vi "Polarisation.vi"(0 "VISA resource name":refnum<visa-resource-name>, 3 "Shutter Ctrls 2":refnum<vi>, 6 "Shutter on?":bool, 7 "ESP301 Error":errorcluster, 8 "LightField Automation in":refnum<class "LightField Automation.lvclass">, 9 "RotStage Exc Angle Refnum":refnum<vi>, 10 "KCube Shutter Device Reference 2":refnum<vi>, 11 "StopPolar 2":refnum<vi>, 12 "CCD 1D Spectrum Main 3":refnum<vi>, 13 "LightField error":errorcluster, 14 "Polar Params SubVI":T2, 15 "PausePolar":refnum<vi>, 17 "Axis ESP301 / RotStage":u16(ring) items=["RotStage Detection"=2, "RotStage Excitation"=3], 21 "IntGraph Refnum":refnum<vi>, 24 "Slide Refnum":refnum<vi>) -> (2 "KCube Shutter Device Reference":refnum<k24>, 18 "Angles":dbl[](array[numeric]), 19 "Wavelengths":dbl[](array[numeric]), 20 "VISA resource name out":refnum<visa-resource-name>, 23 "LightField Automation out":refnum<class "LightField Automation.lvclass">, 25 "LightField error out":errorcluster, 26 "2D Pol Data":dbl[][](array[numeric]), 27 "ESP301 Error out":errorcluster)   [LabVIEW 2019]
uses:
  Light Field/lightfield-automation-labview/LightField Automation.lvclass
  TypeDefs/AcqMode.ctl
  D:/Users/manip-thz/Documents/Controle_Manip_2020/Thorlabs.MotionControl.KCube.SolenoidCLI.dll
  Thorlabs.MotionControl.KCube.SolenoidCLI.dll
  Newport/Newport ESP301/Newport ESP301.lvlib
panel:
  in  "Polar mode":u16(ring)=3 caption="Rotate HWP" items=["Excitation"=3, "Detection"=2]
  in  "Previous Button":bool
  in  "StopPolar":bool
  out "CCD 1D Spectrum Main 2":cluster{dbl[], dbl[]}(graph)
  in  "XYGraph Refnum":refnum<vi>
  in  "Acq Mode":T1=enum."Spectrum" caption="Acq mode"
  out "2D Data":dbl[][](array[numeric])
  in  "RotStage Exc Angle (°)":dbl=2.0 caption="Readout (°)" min=-360.0 max=360.0
  out "Position (units)":dbl format="%.6g"
  out "Numeric":i32
  out "Motion Done":bool
  in  "Progress":u8(slide) scale=0.0..100.0
  out "Current angle (°)":dbl
  in  "CCD ROI":T3(ring)
  in  "Exposure time (ms)":dbl=100.0
  in  "Step Angle (°)":dbl=5.0
  in  "End Angle (°)":dbl=180.0
  in  "Start Angle (°)":dbl
types:
  T1 = typedef "AcqMode.ctl" = enum16{"Image", "Spectrum", "APD 1", "APD 2", "APD 1+2"}
  T2 = cluster{"Polar End Angle (°)":dbl, "Polar Start Angle (°)":dbl, "Polar Step Angle (°)":dbl, "Acq Mode":T1, "Polar mode":u16, "Exposure Time (ms)":dbl, "CCD ROI":enum16{"Custom ROI", "Full sensor", "Binned full sensor"}}
  T3 = enum16{"Custom ROI", "Full sensor", "Binned full sensor"}
  T4 = enum16{"Contrast", "Spectre", "Polarisation", "Time Trace", "XY Intensity Map"}
  T5 = cluster{"Image":dbl[][][], "Frame Size":cluster{"F":i32, "Y":i32, "X":i32}}[]
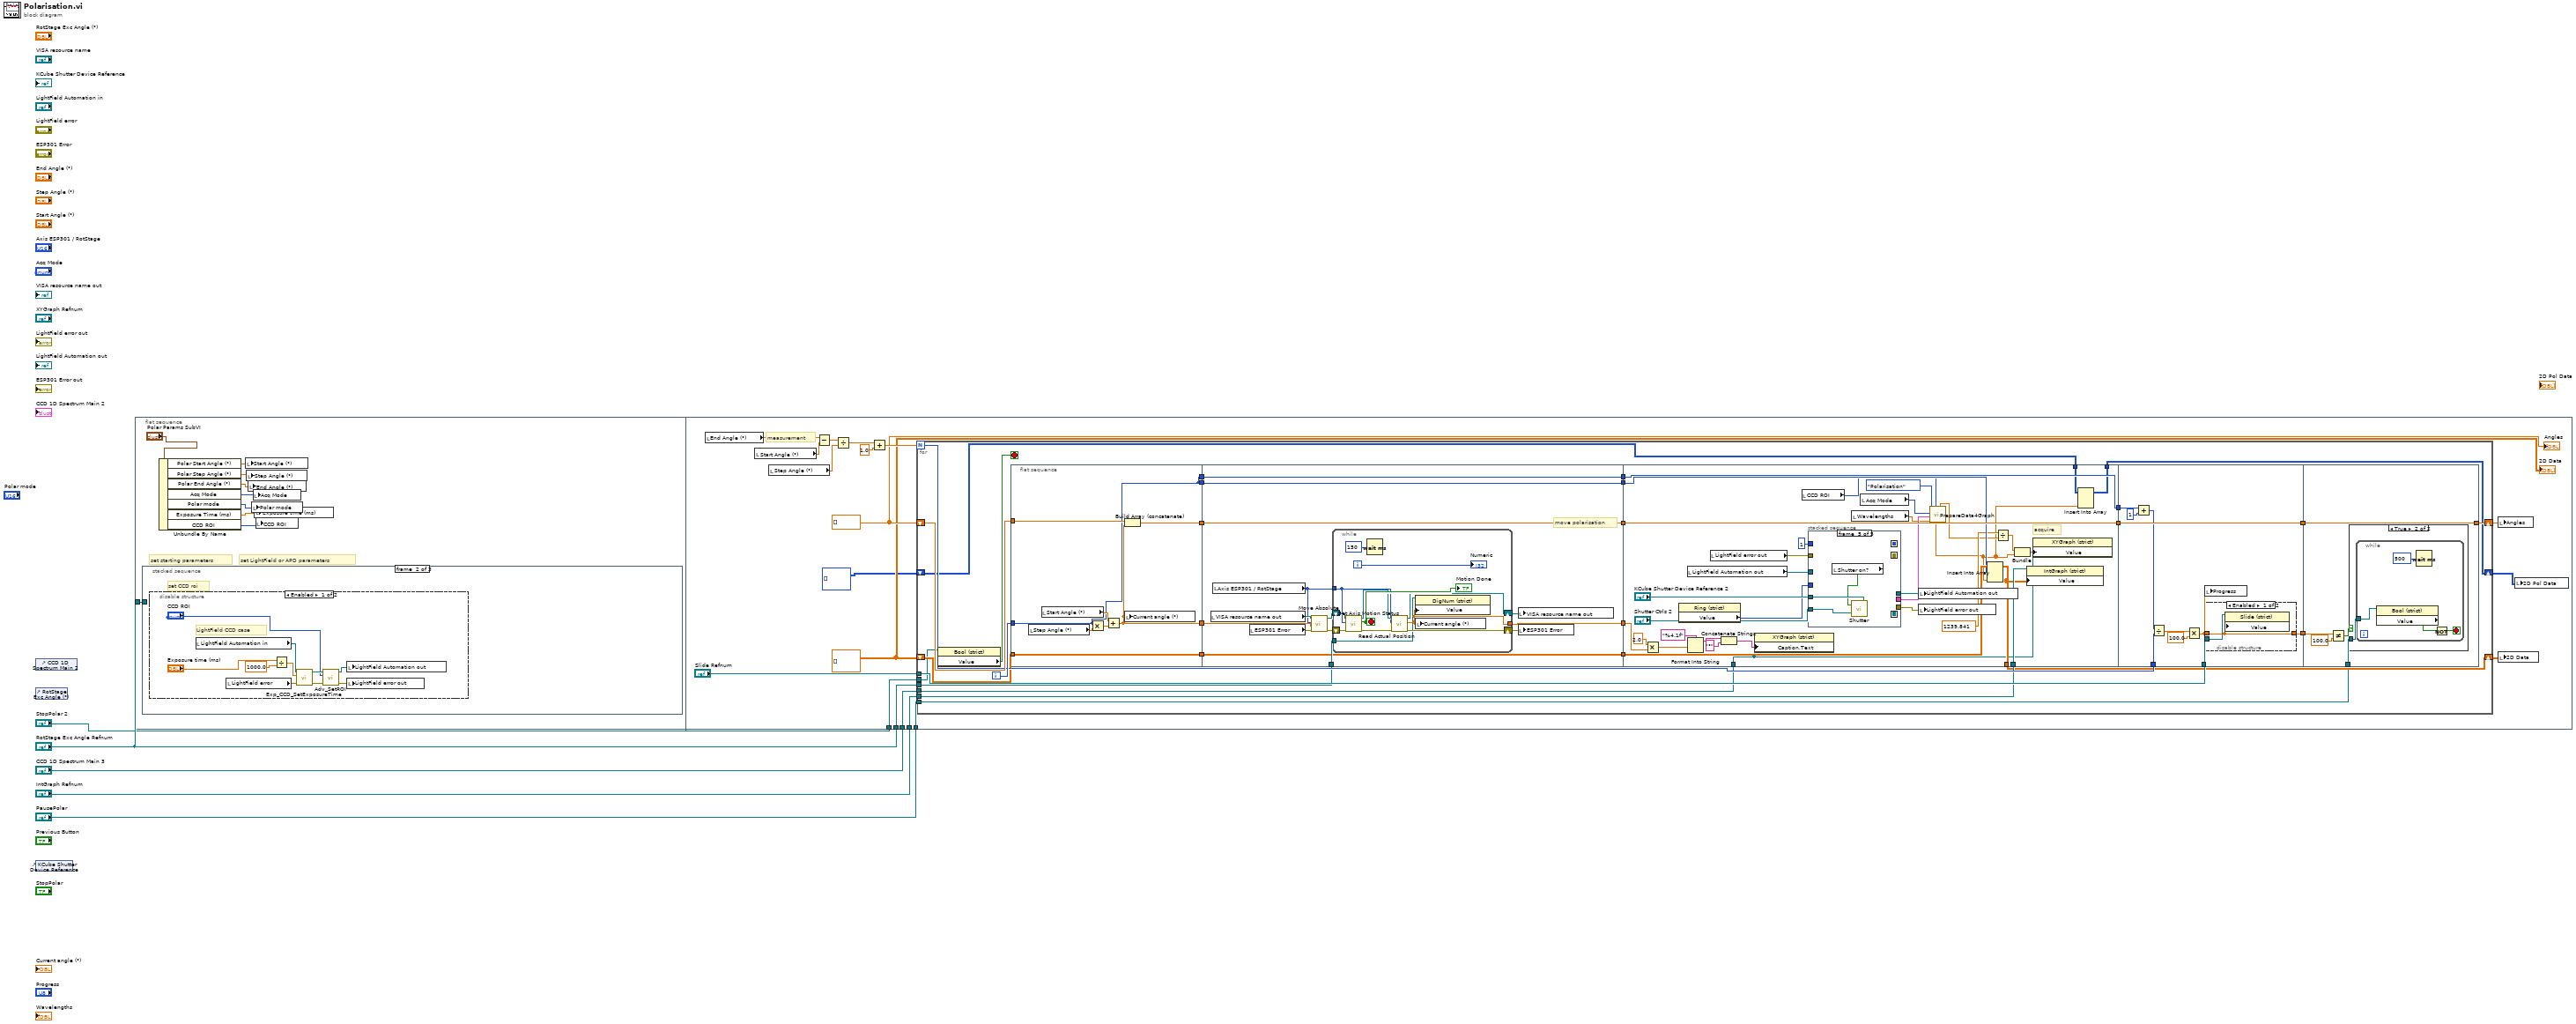
[diagram p0: block diagram]
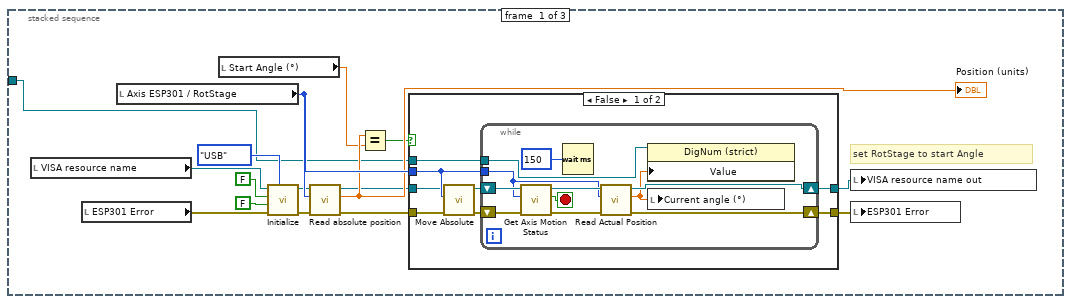
[diagram p2: hidden frame]
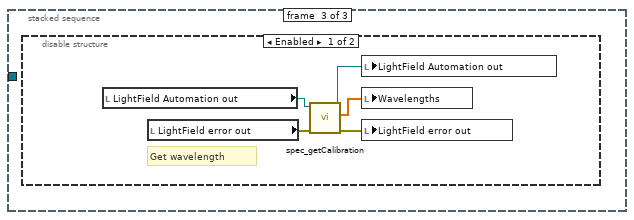
[diagram p5: hidden frame]
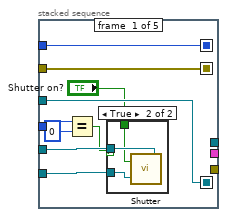
[diagram p7: hidden frame]
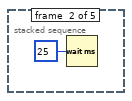
[diagram p9: hidden frame]
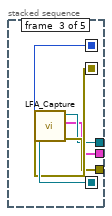
[diagram p10: hidden frame]
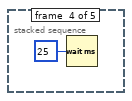
[diagram p11: hidden frame]
diagram:
  n1 = control-ref of="CCD 1D Spectrum Main 2"() -> ()  [unwired: 1 out]
  n2 = control-ref of="RotStage Exc Angle (°)"() -> ()  [unwired: 1 out]
  n3 = control-ref of="KCube Shutter Device Reference"() -> ()  [unwired: 1 out]
  n4 = flat-sequence {
    tunnel: "RotStage Exc Angle Refnum" -> [w14]
    tunnel: "RotStage Exc Angle Refnum" -> [w75]
    tunnel: "IntGraph Refnum" -> [w74]
    tunnel: "CCD 1D Spectrum Main 3" -> [w71]
    tunnel: "StopPolar 2" -> [w70]
    tunnel: "PausePolar" -> [w69]
    frame #0 {
      # "set LightField or APD parameters"
      # "set starting parameters"
      n5 = stacked-sequence {
        tunnel: w14 -> [w15 _ _]
        frame #0 {
          # "set RotStage to start Angle"
          n6 = local read "VISA resource name"() -> (w22:refnum<visa-resource-name>)
          n7 = local read "ESP301 Error"() -> (w16:errorcluster)
          n8 = local read "Axis ESP301 / RotStage"() -> (w28:u16)
          n9 = local read "Start Angle (°)"() -> (w26:dbl)
          n10 = call "Initialize.vi"("VISA resource name"=w22, "ID Query (True)"=FALSE, "Reset (False)"=FALSE, "error in (no error)"=w16, "Serial Link (RS232)"=enum16{"RS232", "USB"}."USB") -> ("VISA resource name out"=w18:refnum<visa-resource-name>, "error out"=w17:errorcluster)  [unwired: 4 in]
          n11 = call "Read absolute position.vi"("error in (no error)"=w17, "Axis (1)"=w28, "VISA resource name"=w18) -> ("error out"=w24:errorcluster, "Position (units)"=w27:dbl, "VISA resource name out"=w23:refnum<visa-resource-name>)  [unwired: 2 in]
          "Position (units)" <- w27
          n12 = Equal?(x=w27, y=w26) -> (x = y?=w25:bool)
          n13 = case shown="False" w25 {
            tunnel: [w38 w51] -> w30
            tunnel: [w37 w50] -> w29
            tunnel: w28 -> [w34 _]
            tunnel: w24 -> [w33 w50]
            tunnel: w23 -> [w32 w51]
            tunnel: w15 -> [w31 _]
            frame False {
              n14 = call "Move Absolute.vi"("error in (no error)"=w33, "Axis (1)"=w34, "VISA resource name"=w32) -> ("error out"=w35:errorcluster, "VISA resource name out"=w36:refnum<visa-resource-name>)  [unwired: 3 in]
              n15 = while {
                tunnel: w34 -> [w43]
                shift-right: [w44] -> w38
                shift-left: w36 -> [w49]
                shift-right: [w41] -> w37
                shift-left: w35 -> [w48]
                tunnel: w31 -> [w39]
                stop <- w47 stop-if-true
                n16 = call "Get Axis Motion Status.vi"("error in (no error)"=w48, "Axis (1)"=w43, "VISA resource name"=w49) -> ("error out"=w42:errorcluster, "Motion Done"=w47:bool, "VISA resource name out"=w45:refnum<visa-resource-name>)  [unwired: 2 in]
                n17 = Wait (ms)(milliseconds to wait=u32 150) -> ()  [unwired: 1 out]
                n18 = call "Read Actual Position.vi"("error in (no error)"=w42, "Axis (1)"=w43, "VISA resource name"=w45) -> ("error out"=w41:errorcluster, "Position (units)"=w40:dbl, "VISA resource name out"=w44:refnum<visa-resource-name>)  [unwired: 2 in]
                n19 = property class="DigNum (strict)"(reference=w39, "Value"=w40) -> ()  [unwired: 1 in, 2 out]
                n20 = local write "Current angle (°)"(w40) -> ()
              }
            }
            frame True {
            }
          }
          n21 = local write "VISA resource name out"(w30) -> ()
          n22 = local write "ESP301 Error"(w29) -> ()
        }
        frame #1 {
          # "set CCD roi"
          n23 = disable-structure shown="Enabled" {
            frame Enabled {
              # "LightField CCD case"
              n24 = local read "LightField Automation in"() -> (w57:refnum<class "LightField Automation.lvclass">)
              n25 = local read "LightField error"() -> (w58:errorcluster)
              n26 = Divide(x="Exposure time (ms)", y=1000.0) -> (x/y=w59:dbl)
              n27 = call "Exp_CCD_SetExposureTime.vi"("error in (no error)"=w58, "Exposure Time (s)"=w59, "LightField Automation in"=w57) -> ("error out"=w55:errorcluster, "LightField Automation out"=w56:refnum<class "LightField Automation.lvclass">)  [unwired: 7 in]
              n28 = call "Adv_SetROI.vi"("error in (no error)"=w55, "ROI"="CCD ROI", "LightField Automation in"=w56) -> ("error out"=w54:errorcluster, "LightField Automation out"=w53:refnum<class "LightField Automation.lvclass">)  [unwired: 7 in]
              n29 = local write "LightField Automation out"(w53) -> ()
              n30 = local write "LightField error out"(w54) -> ()
            }
            frame Disabled {
            }
          }
        }
        frame #2 {
          n31 = disable-structure shown="Enabled" {
            frame Enabled {
              # "Get wavelength"
              n32 = local read "LightField Automation out"() -> (w66:refnum<class "LightField Automation.lvclass">)
              n33 = local read "LightField error out"() -> (w65:errorcluster)
              n34 = call "spec_getCalibration.vi"("error in (no error)"=w65, "LightField Automation in"=w66) -> ("error out"=w63:errorcluster, "ColumnCalibration"=w62:dbl[], "LightField Automation out"=w64:refnum<class "LightField Automation.lvclass">)  [unwired: 7 in]
              n35 = local write "LightField Automation out"(w64) -> ()
              n36 = local write "Wavelengths"(w62) -> ()
              n37 = local write "LightField error out"(w63) -> ()
            }
            frame Disabled {
            }
          }
        }
      }
      n38 = Unbundle By Name("Polar Params SubVI") -> ("Polar Start Angle (°)"=w10:dbl, "Polar Step Angle (°)"=w11:dbl, "Polar End Angle (°)"=w9:dbl, "Acq Mode"=w8:T1, "Polar mode"=w6:u16, "Exposure Time (ms)"=w7:dbl, "CCD ROI"=w12:T3)
      n39 = local write "Start Angle (°)"(w10) -> ()
      n40 = local write "Step Angle (°)"(w11) -> ()
      n41 = local write "End Angle (°)"(w9) -> ()
      n42 = local write "Polar mode"(w6) -> ()
      n43 = local write "Acq Mode"(w8) -> ()
      n44 = local write "Exposure time (ms)"(w7) -> ()
      n45 = local write "CCD ROI"(w12) -> ()
    }
    frame #1 {
      w73 = dbl[][] []
      w76 = dbl[] []
      # "measurement"
      n46 = local read "End Angle (°)"() -> (w78:dbl)
      n47 = local read "Start Angle (°)"() -> (w79:dbl)
      n48 = local read "Step Angle (°)"() -> (w81:dbl)
      n49 = Subtract(x=w78, y=w79) -> (x-y=w80:dbl)
      n50 = Divide(x=w80, y=w81) -> (x/y=w82:dbl)
      n51 = Add(x=w82, y=1.0) -> (x+y=w83:dbl)
      n52 = for {
        N: w83 -> [w110]
        shift-right: [w113] -> w84
        shift-left: w76 -> [w114]
        tunnel: "Slide Refnum" -> [w108]
        tunnel: w75 -> [w102]
        tunnel: w74 -> [w101]
        shift-right: [w97] -> w72
        shift-left: w73 -> [w100]
        tunnel: w71 -> [w94]
        tunnel: w70 -> [w92]
        tunnel: w69 -> [w89]
        shift-right: [w86] -> w67
        shift-left: i32[][] [] -> [w87]
        i -> [w112]
        stop <- w91 stop-if-true
        n53 = property class="Bool (strict)"(reference=w92) -> ("Value"=w91:bool)  [unwired: 1 in, 2 out]
        n54 = flat-sequence {
          tunnel: w114 -> [w122]
          tunnel: w112 -> [w115]
          tunnel: [w121] -> w107
          tunnel: [w115] -> w105
          tunnel: [w117] -> w103
          tunnel: w100 -> [w116]
          tunnel: [w116] -> w98
          tunnel: [w115] -> w96
          tunnel: w107 -> [w136]
          tunnel: [w136] -> w106
          tunnel: w105 -> [w135]
          tunnel: [w135] -> w104
          tunnel: w103 -> [w132]
          tunnel: w102 -> [w126]
          tunnel: [w125] -> w99
          tunnel: w98 -> [w125]
          tunnel: w96 -> [w124]
          tunnel: [w124] -> w95
          tunnel: [w123] -> w93
          tunnel: w106 -> [w179]
          tunnel: [w179] -> w111
          tunnel: [w182] -> w109
          tunnel: w104 -> [w182]
          tunnel: w101 -> [w181]
          tunnel: w99 -> [w180]
          tunnel: [w178] -> w97
          tunnel: w95 -> [w177]
          tunnel: w94 -> [w168]
          tunnel: w93 -> [w158]
          tunnel: w87 -> [w154]
          tunnel: [w153] -> w86
          tunnel: w111 -> [w215]
          tunnel: w110 -> [w212]
          tunnel: w109 -> [w211]
          tunnel: w108 -> [w208]
          tunnel: [w215] -> w90
          tunnel: [w206] -> w88
          tunnel: [w222] -> w113
          tunnel: w90 -> [w222]
          tunnel: w89 -> [w221]
          tunnel: w88 -> [w220]
          frame #0 {
            n55 = local read "Step Angle (°)"() -> (w119:dbl)
            n56 = local read "Start Angle (°)"() -> (w120:dbl)
            n57 = Multiply(x=w115, y=w119) -> (x*y=w118:dbl)
            n58 = Add(x=w120, y=w118) -> (x+y=w117:dbl)
            n59 = Build Array (concatenate)(w122, w117) -> (w121:dbl[])
            n60 = local write "Current angle (°)"(w117) -> ()
          }
          frame #1 {
            # "move polarisation"
            n61 = local read "VISA resource name out"() -> (w134:refnum<visa-resource-name>)
            n62 = local read "Axis ESP301 / RotStage"() -> (w129:u16)
            n63 = local read "ESP301 Error"() -> (w133:errorcluster)
            n64 = call "Move Absolute.vi"("error in (no error)"=w133, "Position (0 units)"=w132, "Axis (1)"=w129, "VISA resource name"=w134) -> ("error out"=w131:errorcluster, "VISA resource name out"=w130:refnum<visa-resource-name>)  [unwired: 2 in]
            n65 = while {
              tunnel: w129 -> [w141]
              shift-right: [w140] -> w127
              shift-left: w130 -> [w146]
              shift-right: [w139] -> w128
              shift-left: w131 -> [w147]
              tunnel: w126 -> [w138]
              tunnel: [w137] -> w123
              i -> [w145]
              stop <- w148 stop-if-true
              n66 = call "Get Axis Motion Status.vi"("error in (no error)"=w147, "Axis (1)"=w141, "VISA resource name"=w146) -> ("error out"=w143:errorcluster, "Motion Done"=w148:bool, "VISA resource name out"=w142:refnum<visa-resource-name>)  [unwired: 2 in]
              "Motion Done" <- w148
              n67 = Wait (ms)(milliseconds to wait=u32 150) -> ()  [unwired: 1 out]
              n68 = call "Read Actual Position.vi"("error in (no error)"=w143, "Axis (1)"=w141, "VISA resource name"=w142) -> ("error out"=w139:errorcluster, "Position (units)"=w137:dbl, "VISA resource name out"=w140:refnum<visa-resource-name>)  [unwired: 2 in]
              n69 = property class="DigNum (strict)"(reference=w138, "Value"=w137) -> ()  [unwired: 1 in, 2 out]
              n70 = local write "Current angle (°)"(w137) -> ()
              "Numeric" <- w145
            }
            n71 = local write "VISA resource name out"(w127) -> ()
            n72 = local write "ESP301 Error"(w128) -> ()
          }
          frame #2 {
            # "acquire"
            n73 = Multiply(x=2.0, y=w158) -> (x*y=w160:dbl)
            n74 = property class="Ring (strict)"(reference="Shutter Ctrls 2") -> ("Value"=w155:u16)  [unwired: 1 in, 2 out]
            n75 = local read "LightField Automation out"() -> (w176:refnum<class "LightField Automation.lvclass">)
            n76 = Format Into String(format string="%4.1f", w160) -> (resulting string=w167:string)  [unwired: 2 in, 1 out]
            n77 = local read "LightField error out"() -> (w175:errorcluster)
            n78 = Concatenate Strings(w167, "°") -> (w165:string)
            n79 = property class="XYGraph (strict)"(reference=w168, "Caption.Text"=w165) -> ()  [unwired: 1 in, 2 out]
            n80 = local read "CCD ROI"() -> (w149:T3)
            n81 = stacked-sequence {
              seq-local: [w191 _ _ _ _] -> [_ _ w201 _ _]
              seq-local: [w190 _ _ _ _] -> [_ _ w200 _ _]
              seq-local: [w189 _ _ _ _] -> [_ _ w196 _ _]
              tunnel: w176 -> [w191 _ _ _ _]
              tunnel: w175 -> [w190 _ _ _ _]
              tunnel: 1 ("Frames") -> [w189 _ _ _ _]
              tunnel: [_ _ w199 _ _] -> w174
              tunnel: [_ _ w198 _ _] -> w173
              tunnel: [_ _ w197 _ _] -> w172
              tunnel: "Shutter Ctrls 2" -> [w187 _ _ _ w205]
              tunnel: "KCube Shutter Device Reference 2" -> [w188 _ _ _ w204]
              tunnel: w155 -> [w186 _ _ _ _]
              frame #0 {
                n82 = Equal?(x=w186, y=u16 0) -> (x = y?=w185:bool)
                n83 = case shown="True" w185 {
                  tunnel: w188 -> [_ w194]
                  tunnel: w187 -> [_ w193]
                  tunnel: "Shutter on?" -> [_ w192]
                  frame False {
                  }
                  frame True {
                    n84 = call "Shutter.vi"("KCube Shutter Device Reference 2"=w194, "Shutter Ctrls 2"=w193, "Shutter on?"=w192) -> ()
                  }
                }
              }
              frame #1 {
                n85 = Wait (ms)(milliseconds to wait=u32 25) -> ()  [unwired: 1 out]
              }
              frame #2 {
                n86 = call "LFA_Capture.vi"("error in (no error)"=w200, "Frames"=w196, "LightField Automation in"=w201) -> ("error out"=w199:errorcluster, "Data"=w197:T5, "LightField Automation out"=w198:refnum<class "LightField Automation.lvclass">)  [unwired: 6 in]
              }
              frame #3 {
                n87 = Wait (ms)(milliseconds to wait=u32 25) -> ()  [unwired: 1 out]
              }
              frame #4 {
                n88 = local read "Shutter on?"() -> (w203:bool)
                n89 = call "Shutter.vi"("KCube Shutter Device Reference 2"=w204, "Shutter Ctrls 2"=w205, "Shutter on?"=w203) -> ()
              }
            }
            n90 = local read "Wavelengths"() -> (w169:dbl[])
            n91 = local read "Acq Mode"() -> (w170:T1)
            n92 = local write "LightField Automation out"(w173) -> ()
            n93 = local write "LightField error out"(w174) -> ()
            n94 = call "PrepareData4Graph.vi"("Wavelength nm"=w169, "DataLF"=w172, "CCD ROI"=w149, "AcqMode"=w170, "Data type"=T4."Polarisation") -> ("Wavelength out"=w152:dbl[], "PLInt out"=w151:dbl[])  [unwired: 2 in, 2 out]
            n95 = Insert Into Array(array=w180, index (row)=w177, new element=w151) -> (w178:dbl[][])  [unwired: 1 in]
            n96 = Divide(x=1239.841, y=w152) -> (x/y=w161:dbl[])
            n97 = Bundle(w161, "PLInt out"=w151) -> (w162:cluster{dbl[], "PLInt out":dbl[]})  [unwired: 1 in]
            n98 = property class="IntGraph (strict)"(reference=w181, "Value"=w178) -> ()  [unwired: 1 in, 2 out]
            n99 = property class="XYGraph (strict)"(reference=w168, "Value"=w162) -> ()  [unwired: 1 in, 2 out]
            n100 = Insert Into Array(array=w154, new element=w151) -> (w153:i32[][])  [unwired: 2 in]
          }
          frame #3 {
            n101 = Add(x=w211, y=1) -> (x+y=w209:i32)
            n102 = Divide(x=w209, y=w212) -> (x/y=w214:dbl)
            n103 = Multiply(x=w214, y=100.0) -> (x*y=w207:dbl)
            n104 = local write "Progress"(w207) -> ()
            n105 = disable-structure shown="Enabled" {
              disable-tunnel: w208 -> [w217 _]
              disable-tunnel: w207 -> [w216 _]
              disable-tunnel: [w216 _] -> w206
              frame Enabled {
                n106 = property class="Slide (strict)"(reference=w217, "Value"=w216) -> ()  [unwired: 1 in, 2 out]
              }
              frame Disabled {
              }
            }
          }
          frame #4 {
            n107 = Not Equal?(x=w220, y=100.0) -> (x != y?=w218:bool)
            n108 = case shown="True" w218 {
              tunnel: w221 -> [_ w223]
              frame False {
              }
              frame True {
                n109 = while {
                  tunnel: w223 -> [w226]
                  stop <- w224 stop-if-true
                  n110 = property class="Bool (strict)"(reference=w226) -> ("Value"=w225:bool)  [unwired: 1 in, 2 out]
                  n111 = Wait (ms)(milliseconds to wait=u32 500) -> ()  [unwired: 1 out]
                  n112 = Not(x=w225) -> (.not. x?=w224:bool)
                }
              }
            }
          }
        }
      }
      n113 = local write "Angles"(w84) -> ()
      n114 = local write "2D Data"(w72) -> ()
      n115 = local write "2D Pol Data"(w67) -> ()
      "Angles" <- w76
      "2D Data" <- w73
    }
  }
